vi "check source version.vi"(4 "error in (no error)":errorcluster) -> (0 "error out":errorcluster, 1 "continue running?":bool, 2 "year":i32)   [LabVIEW 2015]
uses:
  version state.ctl
panel:
  out "version state":T1
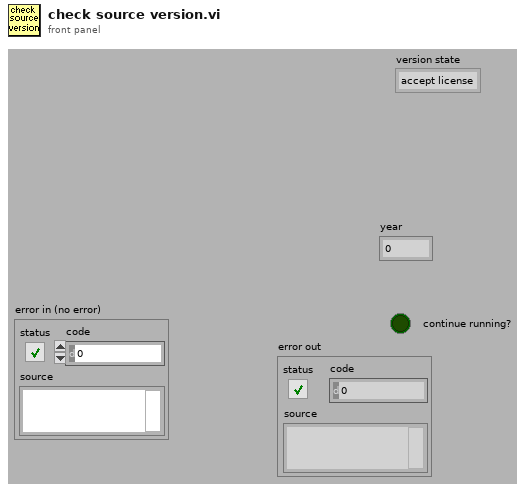
[diagram p1: front panel]
types:
  T1 = typedef "version state.ctl" = enum16{"accept license", "display copyright", "done"}
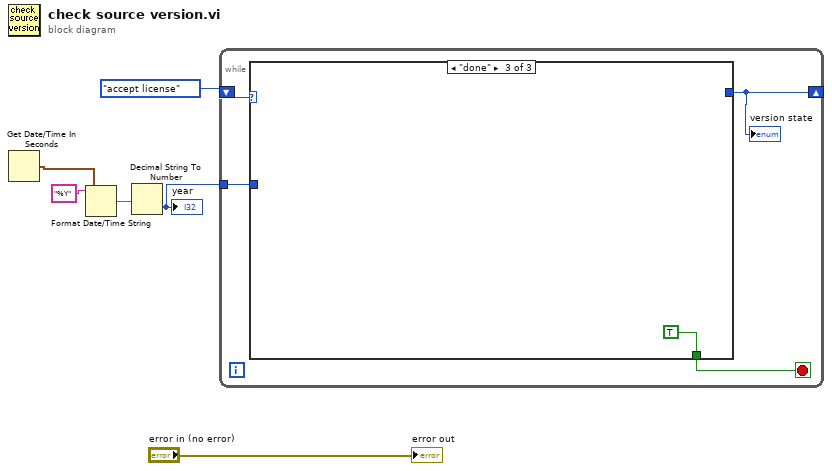
[diagram p0: block diagram]
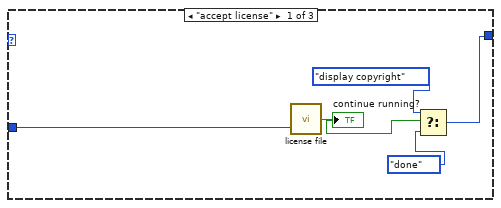
[diagram p2: hidden frame]
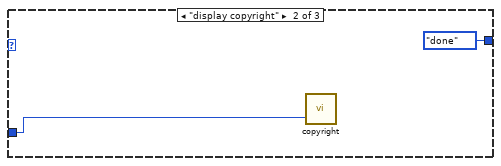
[diagram p3: hidden frame]
diagram:
  n1 = Get Date/Time In Seconds() -> (seconds since 1Jan1904=w2:timestamp)
  n2 = Format Date/Time String(time format string (%c)="%Y", seconds (now)=w2) -> (date/time string=w6:string)  [unwired: 1 in]
  n3 = Decimal String To Number(string=w6) -> (number=w4:i32)  [unwired: 2 in, 1 out]
  "year" <- w4
  n4 = while {
    shift-right: [w10] -> _
    shift-left: version_state."accept license" ("version state") -> [w9]
    tunnel: w4 -> [w8]
    stop <- w7 stop-if-true
    n5 = case shown="\"done\"" w9 {
      tunnel: [w12 version_state."done" ("version state") _] -> w10
      tunnel: w8 -> [w15 w17 _]
      tunnel: [_ _ TRUE] -> w7
      frame "accept license" {
        n6 = call "license file.vi"("year"=w15) -> ("Accepted"=w14:bool)  [unwired: 1 in]
        "continue running?" <- w14
        n7 = Select(t=version_state."display copyright" ("version state"), s=w14, f=version_state."done" ("version state")) -> (s? t:f=w12:T1)
      }
      frame "display copyright" {
        n8 = call "copyright.vi"("year"=w17) -> ()  [unwired: 3 in]
      }
      frame "done" {
      }
    }
    "version state" <- w10
  }
  "error out" <- "error in (no error)"
